vi "Write Refs.vi"(10 "Refs":refnum<class "Refs.lvclass">, 11 "TEMPLATE Actor in":refnum<class "TEMPLATE Actor.lvclass">) -> (3 "TEMPLATE Actor out":refnum<class "TEMPLATE Actor.lvclass">)   [LabVIEW 2020, in "_Template.lvlib" / "Templates.lvlib" / "TEMPLATE jettl Actor.lvlib" / "TEMPLATE Actor.lvlib" / "TEMPLATE Actor.lvclass"]
uses:
  TEMPLATE Actor.lvclass
  jettl/jettl/Refs/Refs.lvclass
  TEMPLATE Actor.lvclass/TEMPLATE Actor.ctl
panel:
  # "This front panel should not be manipulated."
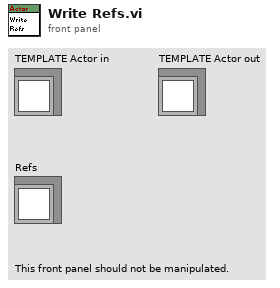
[diagram p1: front panel]
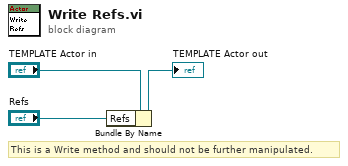
[diagram p0: block diagram]
diagram:
  # "This is a Write method and should not be further manipulated."
  n1 = Bundle By Name(cluster="TEMPLATE Actor in", "Refs"="Refs") -> (→"TEMPLATE Actor out":refnum<class "TEMPLATE Actor.lvclass">)
